vi "Watchdog.vi"() -> ()   [LabVIEW 2018]
uses:
  Data Def/Mitsubishi_Batch Read In Word Units Command.ctl
  Data Def/Mitsubishi_Device Code.ctl
  Data Def/Mitsubishi_Registers Data Type.ctl
  Data Def/Mitsubishi_Batch Write In Word Units Command.ctl
  Data Def/Mitsubishi_Request Message Format.ctl
  Data Def/Mitsubishi_Access Route.ctl
  Data Def/Mitsubishi_Request Type.ctl
panel:
  out "error out":errorcluster
  out "Data":i16(graph)
  out "Cycle Time(ms)":u32
  in  "Stop":bool
  in  "Wait For Writing Time(ms)":u32
  in  "Write Position":T1={"Head Device Number"=0, "Device Code"=168, "Write Data"=[]} {"Write Data" format="%.0x"; "Device Code" items=["SM"=145, "SD"=169, "X*"=156, "Y*"=157, "M*"=144, "L*"=146, "F*"=147, "V*"=148, "B*"=160, "D*"=168, "W*"=180, "TS"=193, "TC"=192, "TN"=194, "SS"=199, "SC"=198, "SN"=200, "CS"=196, "CC"=195, "CN"=197, "SB"=161, "SW"=181, "S*"=152, "DX"=162, "DY"=163, "Z*"=204, "R*"=175, "ZR"=176, "G"=171]}
  in  "Read Position":T3={"Head Device Number"=0, "Device Code"=168, "Number Of Device Point"=1, "Registers Data Type"=enum."16 Bit int"} {"Device Code" items=["SM"=145, "SD"=169, "X*"=156, "Y*"=157, "M*"=144, "L*"=146, "F*"=147, "V*"=148, "B*"=160, "D*"=168, "W*"=180, "TS"=193, "TC"=192, "TN"=194, "SS"=199, "SC"=198, "SN"=200, "CS"=196, "CC"=195, "CN"=197, "SB"=161, "SW"=181, "S*"=152, "DX"=162, "DY"=163, "Z*"=204, "R*"=175, "ZR"=176, "G"=171]}
  out "Read Boolean Data":bool[](array[boolean])
  in  "Port":u16=2000
  in  "IP Address":string="192.168.3.250"
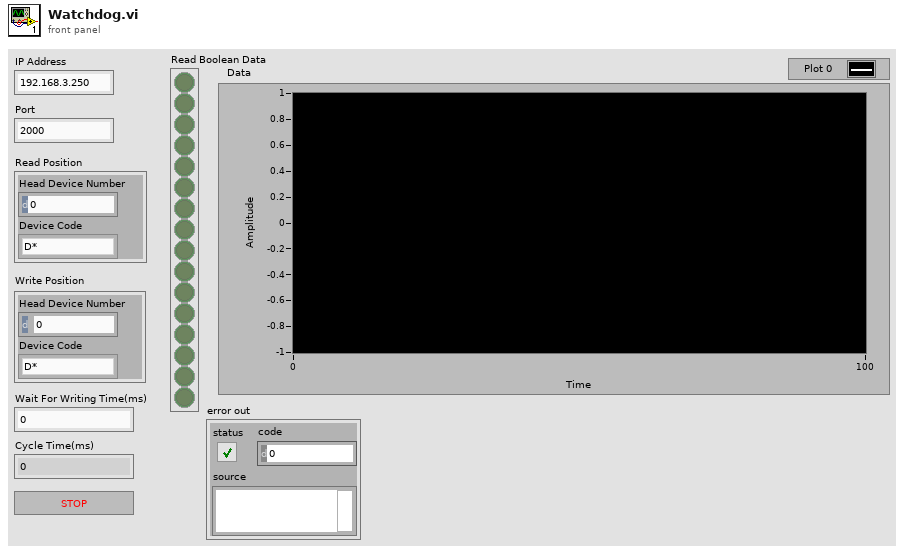
[diagram p1: front panel]
types:
  T1 = typedef "Mitsubishi_Batch Write In Word Units Command.ctl" = cluster{"Head Device Number":u16, "Device Code":T2, "Write Data":i16[]}
  T2 = typedef "Mitsubishi_Device Code.ctl" = u8
  T3 = typedef "Mitsubishi_Batch Read In Word Units Command.ctl" = cluster{"Head Device Number":u16, "Device Code":T2, "Number Of Device Point":u16, "Registers Data Type":T4}
  T4 = typedef "Mitsubishi_Registers Data Type.ctl" = enum16{"16 Bit int", "16 Bit Uint", "32 Bit int", "32 Bit Uint", "32 Bit float", "64 Bit double", "Characters"}
  T5 = enum16{"Standard", "Buffered", "CRLF", "Immediate"}
  T6 = typedef "Mitsubishi_Request Message Format.ctl" = cluster{"Access Route":T7, "Monitoring Timer(ms)":u16, "Request Type":T8, "Request Data":variant}
  T7 = typedef "Mitsubishi_Access Route.ctl" = cluster{"Network No.":string, "PC No.":string, "Module I/O No.":string, "Module Station No.":string}
  T8 = typedef "Mitsubishi_Request Type.ctl" = enum16{"Batch read in word units", "Batch write in word units"}
  T9 = typedef "Mitsubishi_Read Response Message.ctl" = cluster{"Subheader":u16, "Access Route":cluster{"Network No.":u8, "PC No.":u8, "Module I/O No.":u16, "Module Station No.":u8}, "Response Data Length":u8, "End Code":u16, "Response Data":i16[]}
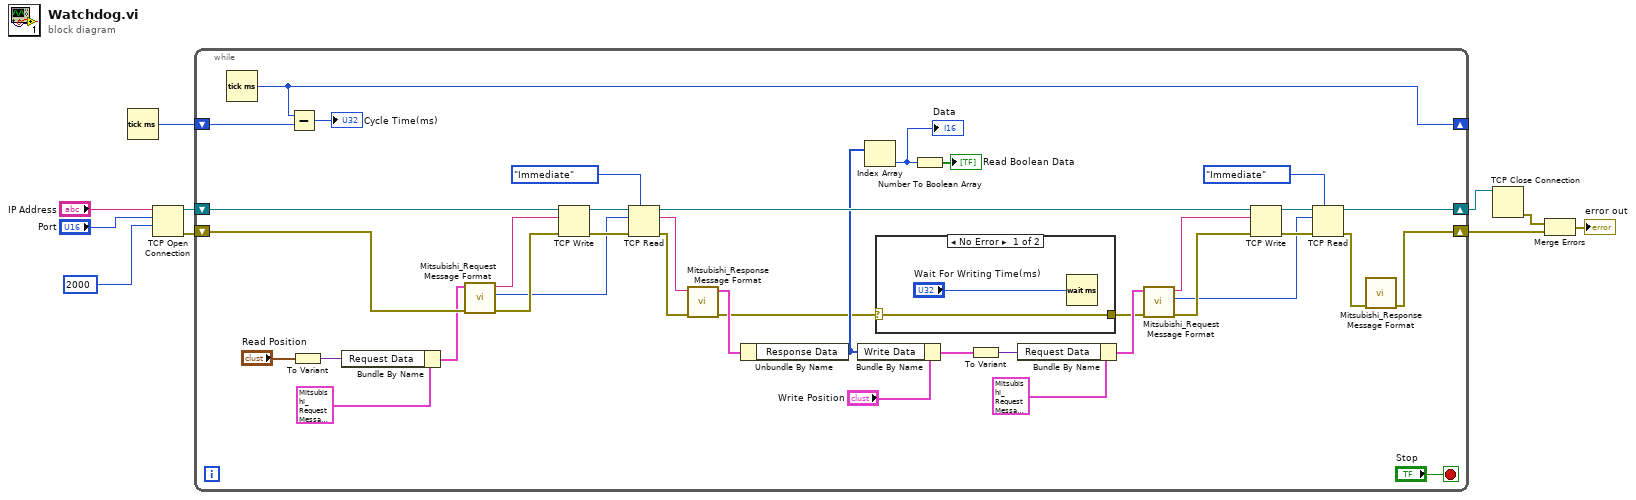
[diagram p0: block diagram]
diagram:
  n1 = Tick Count (ms)() -> (millisecond timer value=w5:u32)
  n2 = TCP Open Connection(address="IP Address", remote port or service name="Port", timeout ms (60000)=2000) -> (connection ID=w7:refnum<k5>, error out=w6:errorcluster)  [unwired: 2 in]
  n3 = while {
    shift-right: [w21] -> w1
    shift-left: w7 -> [w45]
    shift-right: [w20] -> w2
    shift-left: w6 -> [w48]
    shift-right: [w14] -> _
    shift-left: w5 -> [w13]
    stop <- "Stop" stop-if-true
    n4 = Tick Count (ms)() -> (millisecond timer value=w14:u32)
    n5 = Subtract(x=w14, y=w13) -> (x-y=→"Cycle Time(ms)":u32)
    n6 = To Variant(anything="Read Position") -> (Variant=w47:variant)
    n7 = Bundle By Name(cluster=T6 {"Access Route"={"Network No."="\u0000", "PC No."="ÿ", "Module I/O No."="\u0003", "Module Station No."="\u0000"}, "Monitoring Timer(ms)"=4000, "Request Type"=enum."Batch read in word units", "Request Data"=variant} ("Message Format"), "Request Data"=w47) -> (w46:T6)
    n8 = call "Mitsubishi_Request Message Format.vi"("error in"=w48, "Request Message Format"=w46) -> ("error out"=w44:errorcluster, "Byte To Read"=w39:i32, "Request Message"=w43:string)  [unwired: 7 in]
    n9 = TCP Write(connection ID=w45, data in=w43, error in (no error)=w44) -> (connection ID out=w41:refnum<k5>, error out=w42:errorcluster)  [unwired: 1 in, 1 out]
    n10 = TCP Read(connection ID=w41, bytes to read=w39, error in (no error)=w42, 7:T5."Immediate" ("mode (standard)")) -> (connection ID out=w27:refnum<k5>, data out=w37:string, error out=w38:errorcluster)  [unwired: 1 in]
    n11 = call "Mitsubishi_Response Message Format.vi"("error in"=w38, "Respond Data"=w37) -> ("error out"=w17:errorcluster, "Response Message"=w36:T9)  [unwired: 8 in]
    n12 = Unbundle By Name(w36) -> ("Response Data"=w19:i16[])
    n13 = Bundle By Name(cluster="Write Position", "Write Data"=w19) -> (w33:T1)
    n14 = Index Array(array=w19) -> (element=w11:i16)  [unwired: 1 in]
    "Data" <- w11
    n15 = case shown="No Error" w17 {
      selector: w17 -> [w51 w52]
      tunnel: [w51 w52] -> w16
      frame No Error {
        n16 = Wait (ms)(milliseconds to wait="Wait For Writing Time(ms)") -> ()  [unwired: 1 out]
      }
      frame Error {
      }
    }
    n17 = Number To Boolean Array(number=w11) -> (Boolean array=→"Read Boolean Data":bool[])
    n18 = To Variant(anything=w33) -> (Variant=w32:variant)
    n19 = Bundle By Name(cluster=T6 {"Access Route"={"Network No."="\u0000", "PC No."="ÿ", "Module I/O No."="\u0003", "Module Station No."="\u0000"}, "Monitoring Timer(ms)"=4000, "Request Type"=enum."Batch write in word units", "Request Data"=variant} ("Message Format"), "Request Data"=w32) -> (w30:T6)
    n20 = call "Mitsubishi_Request Message Format.vi"("error in"=w16, "Request Message Format"=w30) -> ("error out"=w26:errorcluster, "Byte To Read"=w23:i32, "Request Message"=w25:string)  [unwired: 7 in]
    n21 = TCP Write(connection ID=w27, data in=w25, error in (no error)=w26) -> (connection ID out=w28:refnum<k5>, error out=w24:errorcluster)  [unwired: 1 in, 1 out]
    n22 = TCP Read(connection ID=w28, bytes to read=w23, error in (no error)=w24, 7:T5."Immediate" ("mode (standard)")) -> (connection ID out=w21:refnum<k5>, error out=w22:errorcluster)  [unwired: 1 in, 1 out]
    n23 = call "Mitsubishi_Response Message Format.vi"("error in"=w22) -> ("error out"=w20:errorcluster)  [unwired: 9 in, 1 out]
  }
  n24 = TCP Close Connection(connection ID=w1) -> (error out=w4:errorcluster)  [unwired: 2 in, 1 out]
  n25 = Merge Errors(w4, w2) -> (→"error out":errorcluster)
